vi "SetOutput.vi"(0 "state":T2 items=["[read only]"=-2147483648, "off"=0, "on"=1], 5 "error in":T1) -> (14 "state out":T2 items=["[read only]"=-2147483648, "off"=0, "on"=1], 19 "error out":T1)   [LabVIEW 2016]
doc: "Activates (state = 1) or deactivates (state = 0) all electrical outputs of the ASC500. Activation of the output is necessary prior to many operations such as scanning, zControl or performing a spectroscopy."
uses:
  Controls/Output-Activation_Selection.ctl
  Controls/Error_Out.ctl
  Files_ASC500/DLL/ASC500_RemoteControlV27.dll
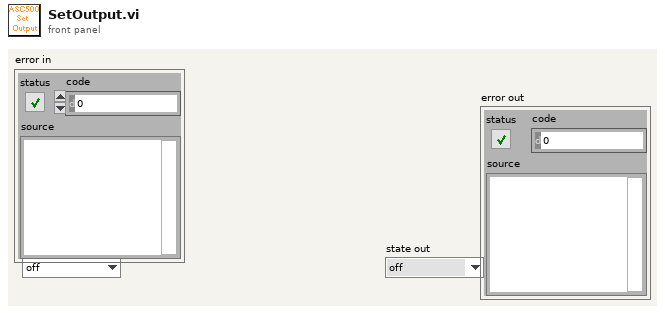
[diagram p1: front panel]
types:
  T1 = typedef "Error_Out.ctl" = errorcluster
  T2 = typedef "Output-Activation_Selection.ctl" = i32
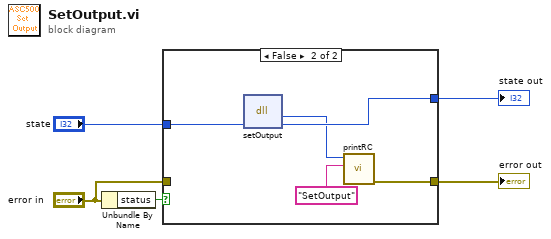
[diagram p0: block diagram]
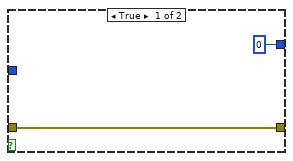
[diagram p2: hidden frame]
diagram:
  n1 = Unbundle By Name("error in") -> ("status"=w5:bool)
  n2 = case shown="False" w5 {
    tunnel: [w6 w10] -> w4
    tunnel: "state" -> [_ w11]
    tunnel: [0 ("State") w12] -> w2
    tunnel: "error in" -> [w6 _]
    frame True {
    }
    frame False {
      n3 = dll-call lib="G:/SCMOperations/Share/ELE/Produkt Information/ASC500/04 Remote Control/02 development versions/2018Nov06/Files_ASC500/DLL/ASC500_RemoteControlV27.dll" fn="setOutput"("State"=w11) -> ("return type"=w9:i32, "State"=w12:i32)  [unwired: 3 in, 2 out]
      n4 = call "printRC.vi"("additional information"="SetOutput", "RC"=w9) -> ("error out"=w10:T1)  [unwired: 9 in]
    }
  }
  "error out" <- w4
  "state out" <- w2
